vi "Main.vi"() -> ()   [LabVIEW 2021]
doc: "The myRIO Project template acquires acceleration data from the onboard accelerometer and displays the changes of acceleration values in a waveform chart."
uses:
  <vilib>/myRIO/Instrument Drivers/Utilities/Utilities.lvlib
  <vilib>/myRIO/Express VI/Onboard Devices/Accelerometer/Accelerometer Express VI.xnode
  <vilib>/myRIO/Instrument Drivers/Onboard Devices/Accelerometer/Accelerometer.lvlib
  <vilib>/myRIO/Common/Instrument Driver Framework/myRIO v1.0/Accelerometer/typedefs/Accelerometer Channels Enum.ctl
  <vilib>/myRIO/Common/Instrument Driver Framework/myRIO v1.0/Accelerometer/typedefs/Accelerometer Channels List.ctl
  <vilib>/myRIO/Common/Instrument Driver Framework/Utilities/typedefs/Generic FPGA Reference.ctl
  <vilib>/myRIO/Common/Instrument Driver Framework/Utilities/typedefs/myRIO v1.0 Reference.ctl
  <vilib>/myRIO/Common/Instrument Driver Framework/Utilities/typedefs/Hardware Version Enum.ctl
  <vilib>/myRIO/Common/Instrument Driver Framework/Utilities/typedefs/myRIO Generic Hardware Reference.ctl
  <vilib>/myRIO/Instrument Drivers/Onboard Devices/Accelerometer/typedefs/Accelerometer Reference.ctl
  <vilib>/myRIO/Instrument Drivers/Onboard Devices/Accelerometer/vis/myRIO Accelerometer Open.xnode
  <vilib>/myRIO/Common/Instrument Driver Framework/Utilities/vis/Is FPGA Ref Available.vi
  <vilib>/myRIO/Common/Instrument Driver Framework/myRIO v1.0/Accelerometer/vis/myRIO v1.1 Open Accelerometer.vi
  <vilib>/userDefined/High Color/nirio_resource_hc.ctl
  <vilib>/myRIO/Instrument Drivers/Onboard IO/UART/typedef/VISA Configuration.ctl
  <vilib>/myRIO/Instrument Drivers/Onboard IO/UART/UART.lvlib
  <vilib>/myRIO/Express VI/Onboard IO/UART/UART Express VI.xnode
  <vilib>/platform/TimedLoop/XDataNode/XDataNode.xnode
  <vilib>/Platform/TimedLoop/XDataNode/nitl_modes.ctl
  <vilib>/Platform/TimedLoop/XDataNode/XDNodeRunTimeDep.lvlib
  <vilib>/Platform/TimedLoop/XDataNode/wakeup.ctl
  <vilib>/Platform/TimedLoop/XDataNode/timing_clust.ctl
  <vilib>/myRIO/Instrument Drivers/Onboard IO/I2C/typedefs/I2C Transfer Rate.ctl
  <vilib>/myRIO/Instrument Drivers/Onboard IO/I2C/I2C.lvlib
  <vilib>/myRIO/Instrument Drivers/Onboard IO/I2C/typedefs/I2C User Configuration.ctl
  <vilib>/myRIO/Instrument Drivers/Onboard IO/I2C/typedefs/I2C Configuration.ctl
  <vilib>/myRIO/Common/Instrument Driver Framework/myRIO v1.0/I2C/typedefs/I2C Channels Enum.ctl
  <vilib>/myRIO/Instrument Drivers/Onboard IO/I2C/typedefs/I2C Reference.ctl
  <vilib>/myRIO/Instrument Drivers/Onboard IO/I2C/vis/Write Read.vi
  <vilib>/myRIO/Common/Instrument Driver Framework/myRIO v1.0/I2C/vis/myRIO v1.1 Open I2C.vi
  <vilib>/myRIO/Instrument Drivers/Onboard IO/I2C/vis/myRIO I2C Open.xnode
  <vilib>/myRIO/Express VI/Onboard IO/I2C/I2C Express VI.xnode
  <vilib>/myRIO/Instrument Drivers/Onboard IO/I2C/vis/Write.vi
  <vilib>/myRIO/Instrument Drivers/Onboard IO/DIO/DIO.lvlib
  <vilib>/Instr/_visa.llb/VISA Configure Serial Port (Instr).vi
  <vilib>/myRIO/Express VI/Onboard IO/SPI/SPI Express VI.xnode
  <vilib>/myRIO/Common/Instrument Driver Framework/myRIO v1.0/DIO/typedefs/DIO Channels Enum.ctl
  <vilib>/myRIO/Common/Instrument Driver Framework/myRIO v1.0/DIO/typedefs/DIO Channels List.ctl
  <vilib>/myRIO/Instrument Drivers/Onboard IO/DIO/typedefs/DIO Reference.ctl
  <vilib>/myRIO/Instrument Drivers/Onboard IO/DIO/vis/Write.vi
  <vilib>/myRIO/Common/Instrument Driver Framework/myRIO v1.0/DIO/vis/myRIO v1.1 Open DIO.vi
  <vilib>/myRIO/Instrument Drivers/Onboard IO/DIO/vis/myRIO DIO Open.xnode
  <vilib>/myRIO/Express VI/Onboard IO/DO/DO Express VI.xnode
  <vilib>/myRIO/Instrument Drivers/Onboard IO/SPI/SPI.lvlib
  <vilib>/myRIO/Instrument Drivers/Onboard IO/SPI/vis/Write Read.vi
  <vilib>/myRIO/Common/Instrument Driver Framework/myRIO v1.0/SPI/typedefs/SPI Frame Length.ctl
  <vilib>/myRIO/Common/Instrument Driver Framework/myRIO v1.0/SPI/typedefs/SPI Data Direction.ctl
  <vilib>/myRIO/Common/Instrument Driver Framework/myRIO v1.0/SPI/typedefs/SPI Clock Polarity.ctl
  <vilib>/myRIO/Common/Instrument Driver Framework/myRIO v1.0/SPI/typedefs/SPI Clock Phase.ctl
  <vilib>/myRIO/Instrument Drivers/Onboard IO/SPI/typedefs/SPI User Configuration.ctl
  <vilib>/myRIO/Instrument Drivers/Onboard IO/SPI/typedefs/SPI Configuration.ctl
  <vilib>/myRIO/Common/Instrument Driver Framework/myRIO v1.0/SPI/typedefs/SPI Channels Enum.ctl
  <vilib>/myRIO/Instrument Drivers/Onboard IO/SPI/typedefs/SPI Reference.ctl
  <vilib>/myRIO/Instrument Drivers/Onboard IO/SPI/vis/myRIO SPI Open.xnode
  <vilib>/myRIO/Common/Instrument Driver Framework/myRIO v1.0/SPI/vis/myRIO v1.1 Open SPI.vi
panel:
  in  "Stop":bool
  out "Light Detection":u8[](array[knob]) scale=0.0..2000.0
  in  "Tree  Warning Dist (<)":u32
  out "Tree Warning":bool
  out "x+y":dbl(slide) scale=0.0..40.0
  out "Alert":bool
  out "Ta":u8[](array[numeric])
  out "Thyst (hysteresis)":u8[](array[numeric]) format="%x"
  out "TSet":u8[](array[numeric]) format="%x"
  out "Config":u8[](array[numeric])
  out "Sonic Distance (in)":u32
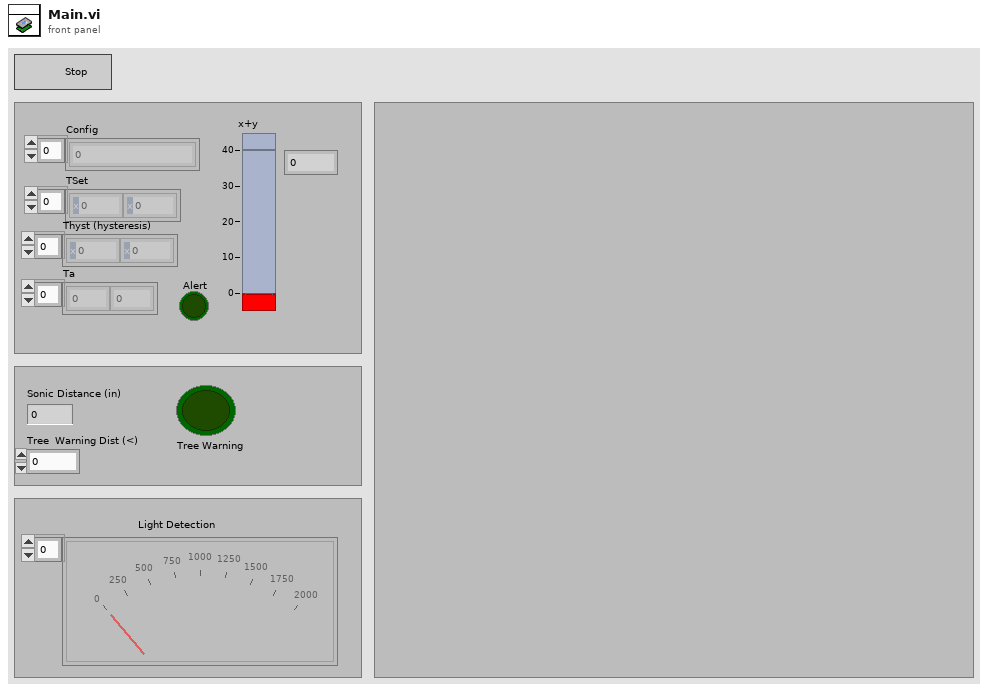
[diagram p1: front panel]
types:
  T1 = typedef "I2C.lvlib/I2C Reference.ctl" = cluster{"myRIO Reference":T2, "I2C Channels Enum":T6, "I2C Configuration":T7}
  T2 = typedef "myRIO Generic Hardware Reference.ctl" = cluster{"myRIO Model":T3, "myRIO Hardware Reference":T4}
  T3 = typedef "Hardware Version Enum.ctl" = enum16{"Unknown", "myRIO-1900", "myRIO-1950", "roboRIO", "NI ELVIS RIO CM", "ELVIS III"}
  T4 = typedef "myRIO v1.0 Reference.ctl" = cluster{"Generic FPGA Reference":T5, "Allow multiple opens":bool}
  T5 = typedef "Generic FPGA Reference.ctl" = refnum<k20>
  T6 = typedef "I2C Channels Enum.ctl" = enum16{"Not Connected", "A/I2C", "B/I2C", "I2C/I2C"}
  T7 = typedef "I2C.lvlib/I2C Configuration.ctl" = cluster{"I2C Transfer Rate":T8}
  T8 = typedef "I2C.lvlib/I2C Transfer Rate.ctl" = enum16{"Standard mode (100 kbps)", "Fast mode (400 kbps)"}
  T9 = typedef "I2C.lvlib/I2C User Configuration.ctl" = cluster{"I2C Transfer Rate":T8}
  T10 = typedef "nirio_resource_hc.ctl" = tag
  T11 = typedef "DIO.lvlib/DIO Reference.ctl" = cluster{"myRIO Reference":T2, "DIO Channels List":T12}
  T12 = typedef "DIO Channels List.ctl" = T13[]
  T13 = typedef "DIO Channels Enum.ctl" = enum16{"Not Connected", "C/DIO0", "C/DIO1", "C/DIO2", "C/DIO3", "C/DIO4", "C/DIO5", "C/DIO6", "C/DIO7", "A/DIO0", "A/DIO1", "A/DIO2", "A/DIO3", "A/DIO4", "A/DIO5", "A/DIO6", "A/DIO7", "A/DIO8", "A/DIO9", "A/DIO10", "A/DIO11", "A/DIO12", "A/DIO13", "A/DIO14", "A/DIO15", "A/DIO16", "A/DIO17", "A/DIO18", "A/DIO19", "B/DIO0", "B/DIO1", "B/DIO2", "B/DIO3", "B/DIO4", "B/DIO5", "B/DIO6", "B/DIO7", "B/DIO8", "B/DIO9", "B/DIO10", "B/DIO11", "B/DIO12", "B/DIO13", "B/DIO14", "B/DIO15", "B/DIO16", "B/DIO17", "B/DIO18", "B/DIO19", "LED0", "LED1", "LED2", "LED3", "Button0", "DIO/DIO0", "DIO/DIO1", "DIO/DIO2", "DIO/DIO3", "DIO/DIO4", "DIO/DIO5", "DIO/DIO6", "DIO/DIO7", "DIO/DIO8", "DIO/DIO9", "SPI/CS0", "SPI/CS1", "SPI/CS2", "SPI/CS3", "LED RADIO (Green)", "LED RADIO (Red)", "LED COMM (Green)", "LED COMM (Red)", "LED MODE (Green)", "LED MODE (Red)"}
  T14 = typedef "SPI.lvlib/SPI Reference.ctl" = cluster{"myRIO Reference":T2, "SPI Channels Enum":T15, "SPI Configuration":T16}
  T15 = typedef "SPI Channels Enum.ctl" = enum16{"Not Connected", "A/SPI", "B/SPI", "SPI/SPI"}
  T16 = typedef "SPI.lvlib/SPI Configuration.ctl" = cluster{"Frequency [Hz]":dbl, "Clock Phase":T17, "Clock Polarity":T18, "Data Direction":T19, "Frame Length":T20}
  T17 = typedef "SPI Clock Phase.ctl" = enum8{"Leading", "Trailing"}
  T18 = typedef "SPI Clock Polarity.ctl" = enum8{"Low", "High"}
  T19 = typedef "SPI Data Direction.ctl" = enum8{"Most significant bit first", "Least significant bit first"}
  T20 = typedef "SPI Frame Length.ctl" = u8
  T21 = typedef "SPI.lvlib/SPI User Configuration.ctl" = cluster{"Frequency [Hz]":dbl, "Clock Phase":T17, "Clock Polarity":T18, "Data Direction":T19, "Frame Length":T20}
  T22 = typedef "XDNodeRunTimeDep.lvlib/timing_clust.ctl" = cluster{"Expected End [f-1]":u64, "Actual End [f-1]":u64, "Finished Late? [f-1]":bool, "Expected End [i-1]":u64, "Actual End [i-1]":u64, "Finished Late? [i-1]":bool, "Expected Start [i]":u64, "Actual Start [i]":u64, "Expected Start [f]":u64, "Actual Start [f]":u64, "Source Name":string, "Structure Name":string, "Period":i64, "Deadline":i64, "Offset":i64, "Start":i64, "Priority":i32, "Timeout":i32, "Mode":T23, "Wakeup Reason":T24, "Error":errorcluster, "Source Type":string, "Secondary Source Type":string, "Global End Time":u64, "Global Start Time":u64, "Frame Duration":u64, "Iteration Duration":u64, "Assigned CPU":i32, "I/O Scan Engine Mode":u32}
  T23 = typedef "XDNodeRunTimeDep.lvlib/nitl_modes.ctl" = enum32{"No Change", "Process missed periods, maintain original phase", "Discard missed periods, maintain original phase", "Process missed periods, ignore original phase", "Discard missed periods, ignore original phase"}
  T24 = typedef "XDNodeRunTimeDep.lvlib/wakeup.ctl" = enum32{"Normal", "Aborted", "Asynchronous wakeup", "Timing source error", "Timed loop error", "Timeout"}
  T25 = typedef "UART.lvlib/VISA Configuration.ctl" = cluster{"baud rate (9600)":u32, "data bits (8)":u16, "parity (0:none)":enum16{"None", "Odd", "Even", "Mark", "Space"}, "stop bits (10: 1 bit)":u16, "flow control (0:none)":u16, "termination char\n(0xA = '\\n' = LF) ":u8, "Enable Termination\nChar (T)":bool, "timeout (10sec)":u32}
  T26 = typedef "Accelerometer.lvlib/Accelerometer Reference.ctl" = cluster{"myRIO Reference":T2, "Accelerometer Channels List":T27, "LSB Weight":dbl}
  T27 = typedef "Accelerometer Channels List.ctl" = T28[]
  T28 = typedef "Accelerometer Channels Enum.ctl" = enum16{"Not Connected", "X-Axis", "Y-Axis", "Z-Axis"}
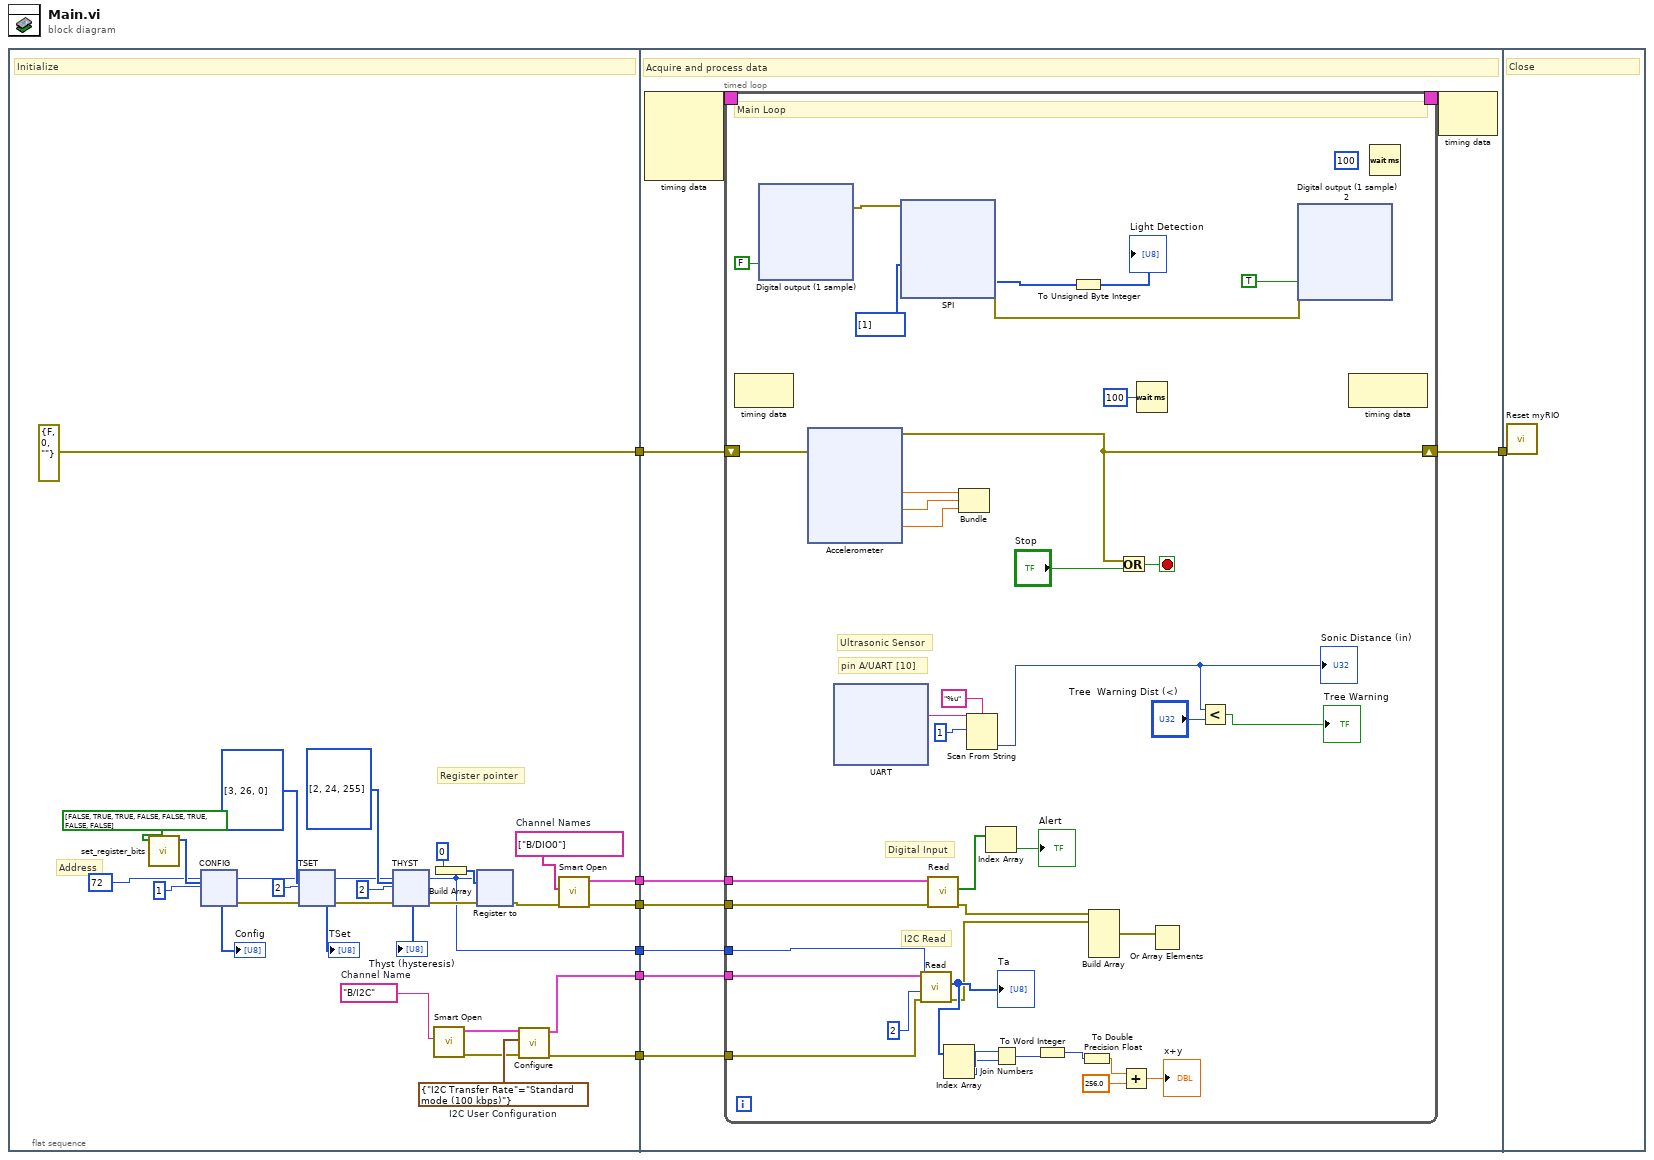
[diagram p0: block diagram]
diagram:
  n1 = flat-sequence {
    tunnel: [errorcluster {"status"=FALSE, "code"=0, "source"=""} ("error in (no error)")] -> w7
    tunnel: [w14] -> w5
    tunnel: [w13] -> w4
    tunnel: [w12] -> w3
    tunnel: [w11] -> w2
    tunnel: [w8] -> w1
    tunnel: w7 -> [w201]
    tunnel: [w200] -> w6
    tunnel: w5 -> [w197]
    tunnel: w4 -> [w196]
    tunnel: w3 -> [w195]
    tunnel: w2 -> [w194]
    tunnel: w1 -> [w193]
    tunnel: w6 -> [w410]
    frame #0 {
      w18 = tag[] ["B/DIO0"]  # Channel Names
      w21 = T9 {"I2C Transfer Rate"=enum."Standard mode (100 kbps)"}  # I2C User Configuration
      w22 = tag "B/I2C"  # Channel Name
      w8 = u8 72 ("Slave Address (7-bit)")
      # "Address"
      # "Register pointer"
      # "Initialize"
      n2 = call "set_register_bits.vi"("Array in"=bool[] [FALSE, TRUE, TRUE, FALSE, FALSE, TRUE, FALSE, FALSE]) -> ("Array out"=w32:u8[])  [unwired: 10 in]
      n3 = xnode "CONFIG"("Slave Address (7-bit)"=w8, "Bytes to Write"=w32, "Byte Count"=u32 1) -> ("error out"=w27:errorcluster, "Bytes Read"=→"Config":u8[])  [unwired: 1 in]
      n4 = xnode "TSET"("error in (no error)"=w27, "Slave Address (7-bit)"=w8, "Bytes to Write"=u8[] [3, 26, 0], "Byte Count"=u32 2) -> ("error out"=w26:errorcluster, "Bytes Read"=→"TSet":u8[])
      n5 = xnode "THYST"("error in (no error)"=w26, "Slave Address (7-bit)"=w8, "Bytes to Write"=u8[] [2, 24, 255], "Byte Count"=u32 2) -> ("error out"=w25:errorcluster, "Bytes Read"=→"Thyst (hysteresis)":u8[])
      n6 = call <vilib>:"Smart Open.vi"("Channel Name"=w22) -> ("error out"=w19:errorcluster, "I2C Ref Out"=w20:T1)  [unwired: 9 in]
      n7 = Build Array(0) -> (w10:i32[])
      n8 = xnode "Register to"("error in (no error)"=w25, "Slave Address (7-bit)"=w8, "Bytes to Write"=w10) -> ("error out"=w17:errorcluster)
      n9 = call <vilib>:"Configure.vi"("error in (no error)"=w19, "I2C User Configuration"=w21, "I2C Ref In"=w20) -> ("error out"=w13:errorcluster, "I2C Ref Out"=w14:T1)  [unwired: 7 in]
      n10 = call <vilib>:"Smart Open.vi"("error in (no error)"=w17, "Channel Names"=w18) -> ("error out"=w11:errorcluster, "DIO Ref Out"=w12:T11)  [unwired: 8 in]
    }
    frame #1 {
      # "Acquire and process data"
      n11 = node-c288() -> (w199:T22)  [unwired: 4 in]
      n12 = timed-loop {
        shift-right: [w237] -> w200
        shift-left: w201 -> [w238]
        timing: w199 -> [_]
        timing-out: [_] -> w198
        tunnel: w197 -> [w220]
        tunnel: w196 -> [w219]
        tunnel: w195 -> [w218]
        tunnel: w194 -> [w217]
        tunnel: w193 -> [w216]
        stop <- w240 stop-if-true
        (unwired) u32 100 ("milliseconds to wait")
        # "I2C Read"
        # "Digital Input"
        # "Ultrasonic Sensor"
        # "pin A/UART [10]"
        # "Main Loop"
        n13 = node-c288() -> ()  [unwired: 1 in, 1 out]
        n14 = xnode "Digital output (1 sample)"("A/DIO2 (Pin 15)"=FALSE) -> ("error out"=w208:errorcluster)  [unwired: 1 in]
        n15 = xnode "Accelerometer"("error in (no error)"=w238) -> ("X-Axis"=w236:dbl, "Y-Axis"=w235:dbl, "Z-Axis"=w234:dbl, "error out"=w237:errorcluster)
        n16 = xnode "UART"() -> ("Characters Read"=w231:string)  [unwired: 1 in, 1 out]
        n17 = xnode "SPI"("Frames to Write"=u16[] [1], "error in (no error)"=w208) -> ("Frames Read"=w206:u16[], "error out"=w207:errorcluster)
        n18 = call <vilib>:"Read.vi"("error in (no error)"=w219, "Byte Count"=u32 2, "Slave Address (7-bit)"=w216, "I2C Ref In"=w220) -> ("error out"=w214:errorcluster, "Bytes Read"=w227:u8[])  [unwired: 4 in, 1 out]
        "Ta" <- w227
        n19 = call <vilib>:"Read.vi"("error in (no error)"=w217, "DIO Ref In"=w218) -> ("error out"=w215:errorcluster, "Values"=w229:bool[])  [unwired: 7 in, 1 out]
        n20 = Index Array(array=w227) -> (element #1=w226:u8, element #2=w225:u8)  [unwired: 2 in]
        n21 = Bundle("X-Axis"=w236, "Y-Axis"=w235, "Z-Axis"=w234) -> ()  [unwired: 1 in, 1 out]
        n22 = Scan From String(format string="%u", input string=w231, initial scan location=u32 1) -> (output 1=w211:u32)  [unwired: 2 in, 3 out]
        "Sonic Distance (in)" <- w211
        n23 = Index Array(array=w229) -> (element=→"Alert":bool)  [unwired: 1 in]
        n24 = Join Numbers(hi=w226, lo=w225) -> ((hi.lo)=w224:u16)
        n25 = To Word Integer(number=w224) -> (16bit integer=w223:i16)
        n26 = To Unsigned Byte Integer(number=w206) -> (unsigned 8bit integer=→"Light Detection":u8[])
        n27 = To Double Precision Float(number=w223) -> (double precision float=w222:dbl)
        n28 = Build Array(w215, w214) -> (w212:errorcluster[])  [unwired: 4 in]
        n29 = Or(x=w237, y="Stop") -> (x .or. y?=w240:bool)
        n30 = Add(x=w222, y=256.0) -> (x+y=→"x+y":dbl)
        n31 = Wait (ms)(milliseconds to wait=u32 100) -> ()  [unwired: 1 out]
        n32 = Or Array Elements(Boolean array=w212) -> ()  [unwired: 1 out]
        n33 = Less?(x=w211, y="Tree  Warning Dist (<)") -> (x < y?=→"Tree Warning":bool)
        n34 = xnode "Digital output (1 sample) 2"("A/DIO2 (Pin 15)"=TRUE ("A/DIO0 (Pin 11)"), "error in (no error)"=w207) -> ()  [unwired: 1 out]
        n35 = node-c288() -> ()  [unwired: 1 in, 1 out]
        n36 = Wait (ms)() -> ()  [unwired: 1 in, 1 out]
      }
      n37 = node-c288(w198) -> ()  [unwired: 1 out]
    }
    frame #2 {
      # "Close"
      n38 = call <vilib>:"Reset myRIO.vi"("error in (no error)"=w410) -> ()  [unwired: 10 in, 1 out]
    }
  }
